vi "Read Message Definition File.vi"(8 "error in (no error)":errorcluster, 11 "Messages Definitions File":path) -> (0 "error out":errorcluster, 3 "Messages":T1[](array[typedef]))   [LabVIEW 2021, in "HMI Messages.lvclass"]
uses:
  HMI Messages.lvclass
  HMI Messages.lvclass/HMI Messages.ctl
  Message Definition.ctl
  <userlib>/_OpenG.lib/string/string.llb/openg_string.lvlib
  <userlib>/_OpenG.lib/file/file.llb/openg_file.lvlib
  <userlib>/_OpenG.lib/file/file.llb/File Exists - Scalar__ogtk.vi
panel:
  out "text":string[](array[string])
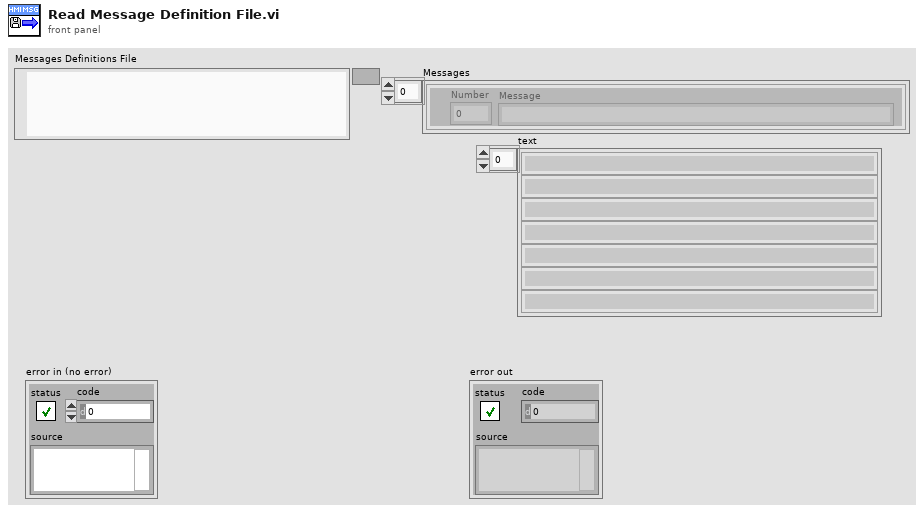
[diagram p1: front panel]
types:
  T1 = typedef "HMI Messages.lvclass/Message Definition.ctl" = cluster{"Number":i32, "Message":string}
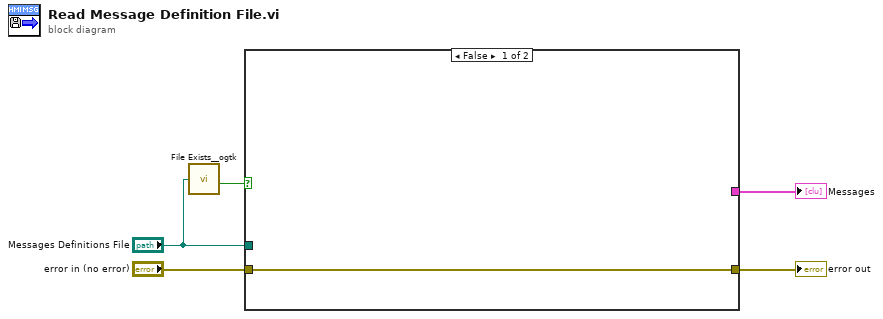
[diagram p0: block diagram]
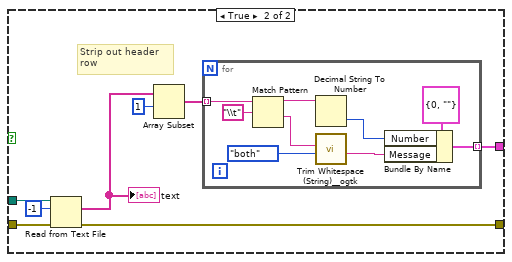
[diagram p2: hidden frame]
diagram:
  n1 = call-poly <userlib>:"File Exists__ogtk.vi"("file path"="Messages Definitions File") -> ("exists"=w1:bool)  [unwired: 6 in, 1 out]
  n2 = case shown="False" w1 {
    tunnel: "error in (no error)" -> [w6 w14]
    tunnel: [w6 w12] -> w4
    tunnel: [_ w11] -> w3
    tunnel: "Messages Definitions File" -> [_ w7]
    frame False {
    }
    frame True {
      # "Strip out header row"
      n3 = Read from Text File(file (use dialog)=w7, count=-1, error in=w14) -> (text=w9:string[], error out=w12:errorcluster)  [unwired: 1 in, 2 out]
      "text" <- w9
      n4 = Array Subset(array=w9, index=1) -> (w8:string[])  [unwired: 1 in]
      n5 = for {
        tunnel: w8 -> [w21] mode=indexing
        tunnel: [w22] -> w11 mode=indexing
        n6 = Match Pattern(string=w21, regular expression="\\t") -> (before substring=w20:string, after substring=w17:string)  [unwired: 1 in, 2 out]
        n7 = Decimal String To Number(string=w20) -> (number=w19:i32)  [unwired: 2 in, 1 out]
        n8 = call <userlib>:"Trim Whitespace (String)__ogtk.vi"("Remove (leading and trailing)"=enum16{"leading", "trailing", "both"}."both", "String in"=w17) -> ("String out"=w16:string)  [unwired: 5 in]
        n9 = Bundle By Name(cluster=T1 {"Number"=0, "Message"=""} ("Message Definition"), "Number"=w19, "Message"=w16) -> (w22:T1)
      }
    }
  }
  "error out" <- w4
  "Messages" <- w3
